vi "VAJ_route_queue.vi"(7 "set":enum16{"reset", "write"}(ring), 11 "move in":T1[](array[typedef])) -> (3 "s? t:f":T1[](array[typedef]))   [LabVIEW 2019]
uses:
  move cluster(VAJ).ctl
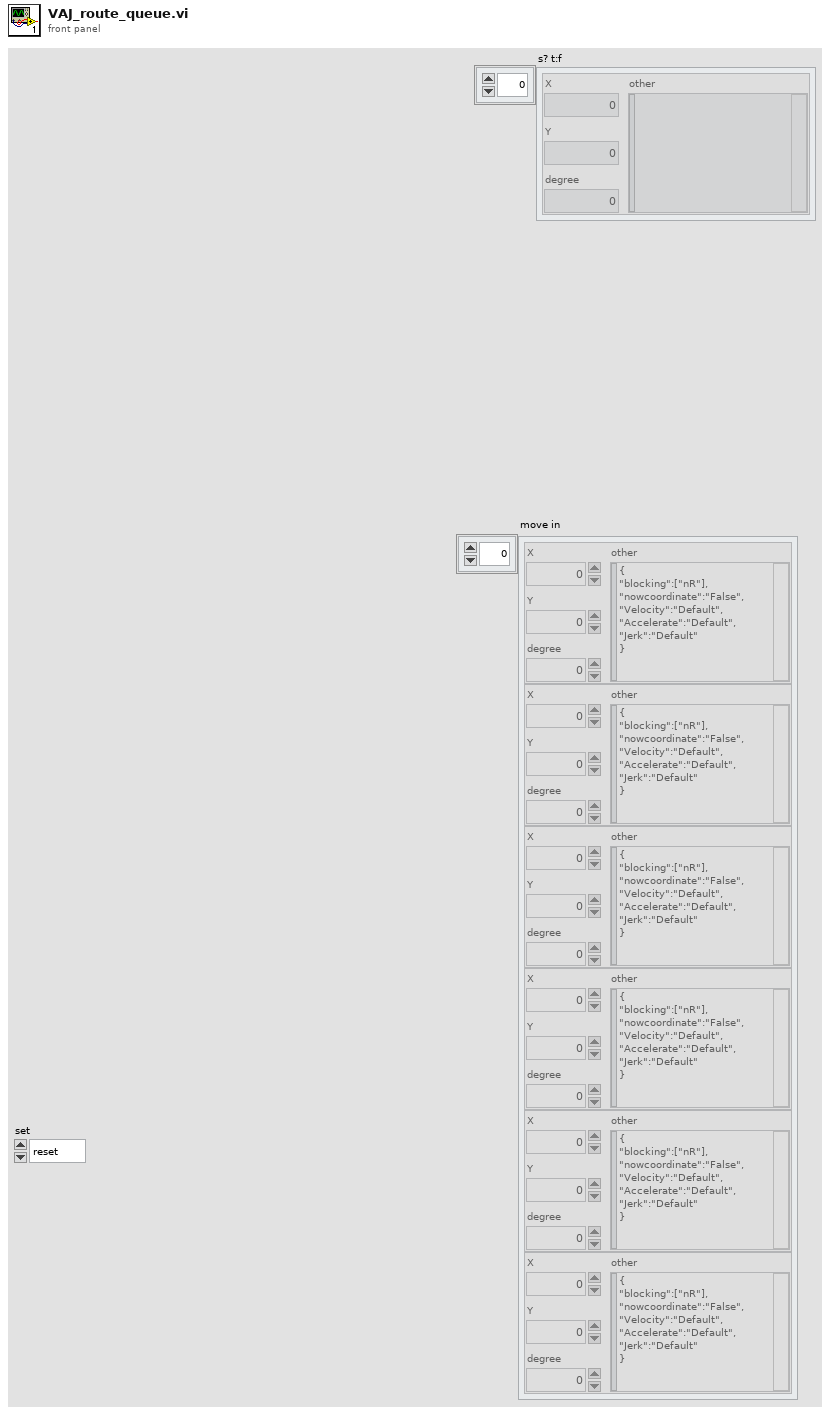
[diagram p1: front panel]
types:
  T1 = typedef "move cluster(VAJ).ctl" = cluster{"X":dbl, "Y":dbl, "degree":dbl, "other":string}
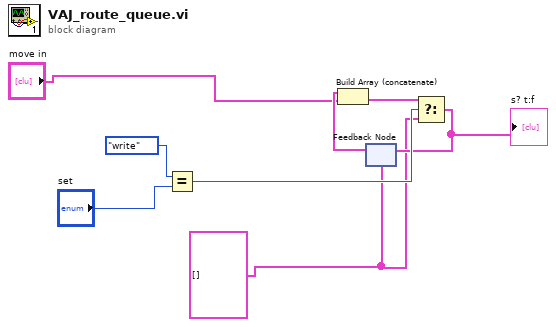
[diagram p0: block diagram]
diagram:
  w1 = T1[] [] ("move in")
  n1 = Equal?(x=enum16{"reset", "write"}."write" ("Enum"), y="set") -> (x = y?=w5:bool)
  n2 = feedback #1(w1) -> (w7:T1[])
  n3 = Build Array (concatenate)(w7, "move in") -> (w4:T1[])
  n4 = Select(t=w4, s=w5, f=w1) -> (s? t:f=w3:T1[])
  "s? t:f" <- w3
  n5 = feedback-in #1(w3) -> ()
